vi "Exp no 3.vi"() -> ()   [LabVIEW 2010]
panel:
  out "X XNOR Y":bool
  out "X XOR Y":bool
  out "X NOR Y":bool
  out "X NAND Y":bool
  out "NOT X":bool
  out "X OR Y":bool
  out "X AND Y":bool
  in  "Boolean Y":bool
  in  "Boolean X":bool
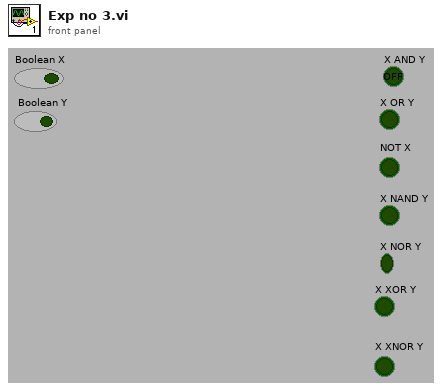
[diagram p1: front panel]
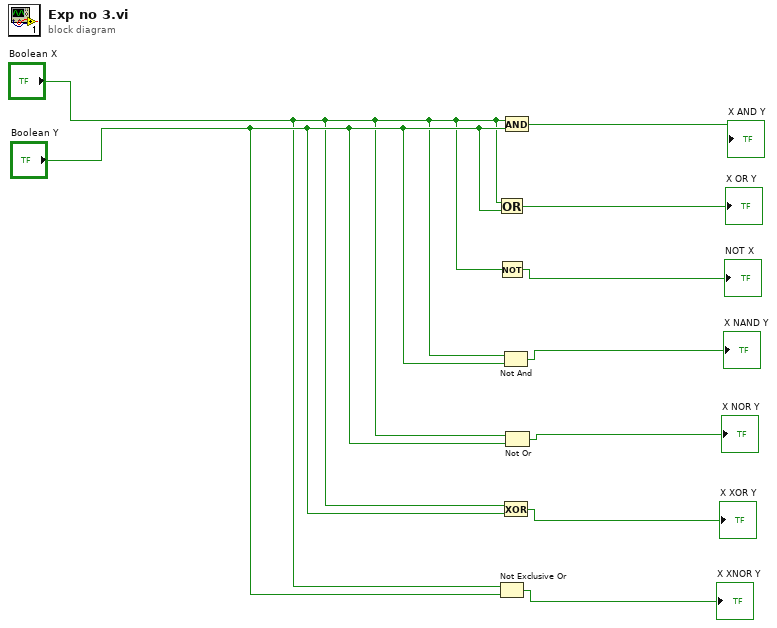
[diagram p0: block diagram]
diagram:
  n1 = Or(x="Boolean X", y="Boolean Y") -> (x .or. y?=→"X OR Y":bool)
  n2 = Not(x="Boolean X") -> (.not. x?=→"NOT X":bool)
  n3 = Not Exclusive Or(1:"Boolean Y", 2:"Boolean X") -> (0:→"X XNOR Y":bool)
  n4 = Not And(1:"Boolean Y", 2:"Boolean X") -> (0:→"X NAND Y":bool)
  n5 = Exclusive Or(1:"Boolean Y", 2:"Boolean X") -> (0:→"X XOR Y":bool)
  n6 = And(x="Boolean X", y="Boolean Y") -> (x .and. y?=→"X AND Y":bool)
  n7 = Not Or(1:"Boolean Y", 2:"Boolean X") -> (0:→"X NOR Y":bool)
